vi "CodigoLabView 3.5.vi"() -> (11 "Releb 2":bool)   [LabVIEW 2025]
uses:
  <vilib>/Utility/NIReport.llb/Report Type.ctl
  <vilib>/Instr/_visa.llb/VISA Configure Serial Port (Instr).vi
  <vilib>/addons/_office/excel.llb/Excel Easy Table (str).vi
  <vilib>/Utility/NIReport.llb/NI_report.lvclass
  <vilib>/addons/_office/NI_ReportGenerationToolkit.lvlib
  <vilib>/Utility/NIReport.llb/NI_ReportGenerationCore.lvlib
  <vilib>/Utility/NIReport.llb/Excel/NI_Excel.lvclass
panel:
  out "errorout":errorcluster
  out "Vrno":refnum<visa-resource-name>
  out "Texto":path=path "C:/Users/Lucas Navarro/Desktop/Ruka/ME2/pf/Jamon.txt"
  out "Historial Tensión de Línea":dbl[](graph)
  out "Historial Tomacorriente 4":dbl[](graph)
  out "Historial Tomacorriente 3":dbl[](graph)
  out "Historial Tomacorriente 2":dbl[](graph)
  out "Historial Tomacorriente 1":dbl[](graph)
  in  "?":bool
  in  "RUTA DE REGISTRO":path
  out "NP4":dbl(knob) scale=0.0..100.0
  out "NP3":dbl(knob) scale=0.0..100.0
  out "NP2":dbl(knob) scale=0.0..100.0
  out "R ON 4":bool
  out "R ON 3":bool
  out "R ON 2":bool
  out "ST":string
  out "R ON 1":bool
  out "NT":dbl(knob) scale=100.0..300.0
  out "NP1":dbl(knob) scale=0.0..100.0
  out "Releb 4":bool
  out "Relea 4":bool
  out "Rele 4":bool
  out "T4":bool
  out "Estado 4":string
  in  "Relé N°4":bool
  out "SP4":string
  out "Releb 3":bool
  out "Relea 3":bool
  out "Rele 3":bool
  out "T3":bool
  out "Estado 3":string
  out "SP3":string
  in  "Relé N°3":bool
  out "Relea 2":bool
  out "Rele 2":bool
  out "T2":bool
  out "Estado 2":string
  out "SP2":string
  in  "Relé N°2":bool
  out "Releb 1":bool
  out "Relea 1":bool
  out "Rele 1":bool
  out "T1":bool
  out "Estado 1":string
  out "SP1":string
  in  "Relé N°1":bool
  in  "PUERTO DE COMUNICACIÓN":refnum<visa-resource-name>
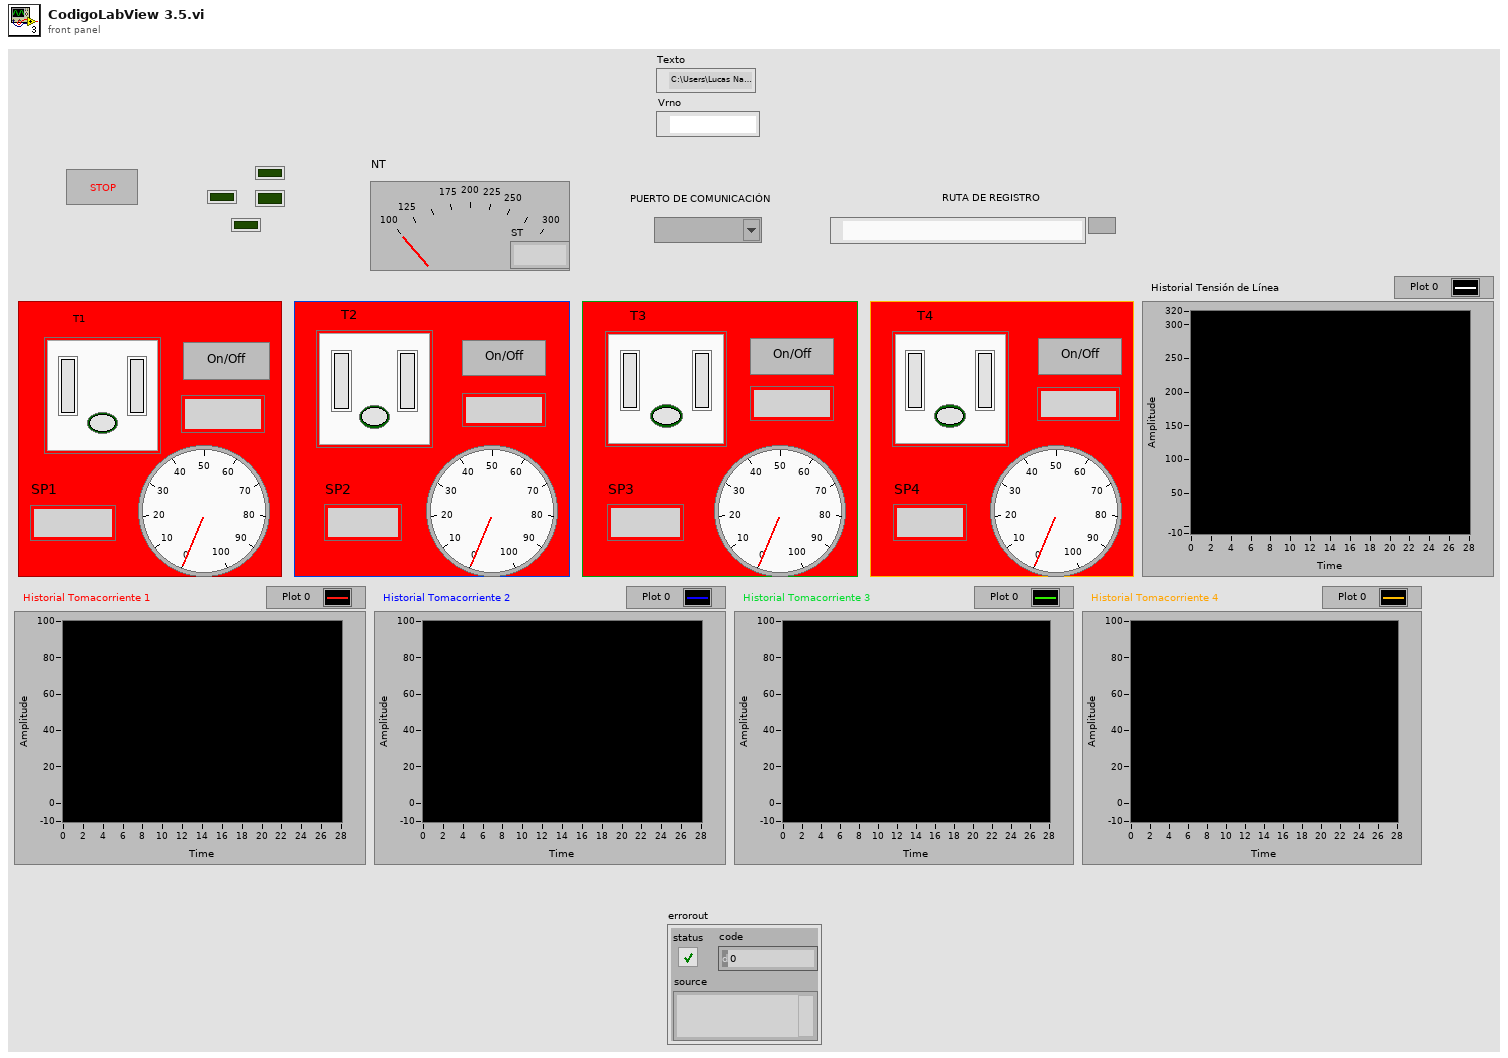
[diagram p1: front panel]
types:
  T1 = typedef "NI_ReportGenerationCore.lvlib/Report Type.ctl" = enum16{"HTML", "Word", "Excel"}
  T2 = cluster{"W1":string, "W2":string, "W3":string, "W4":string, "V":string}
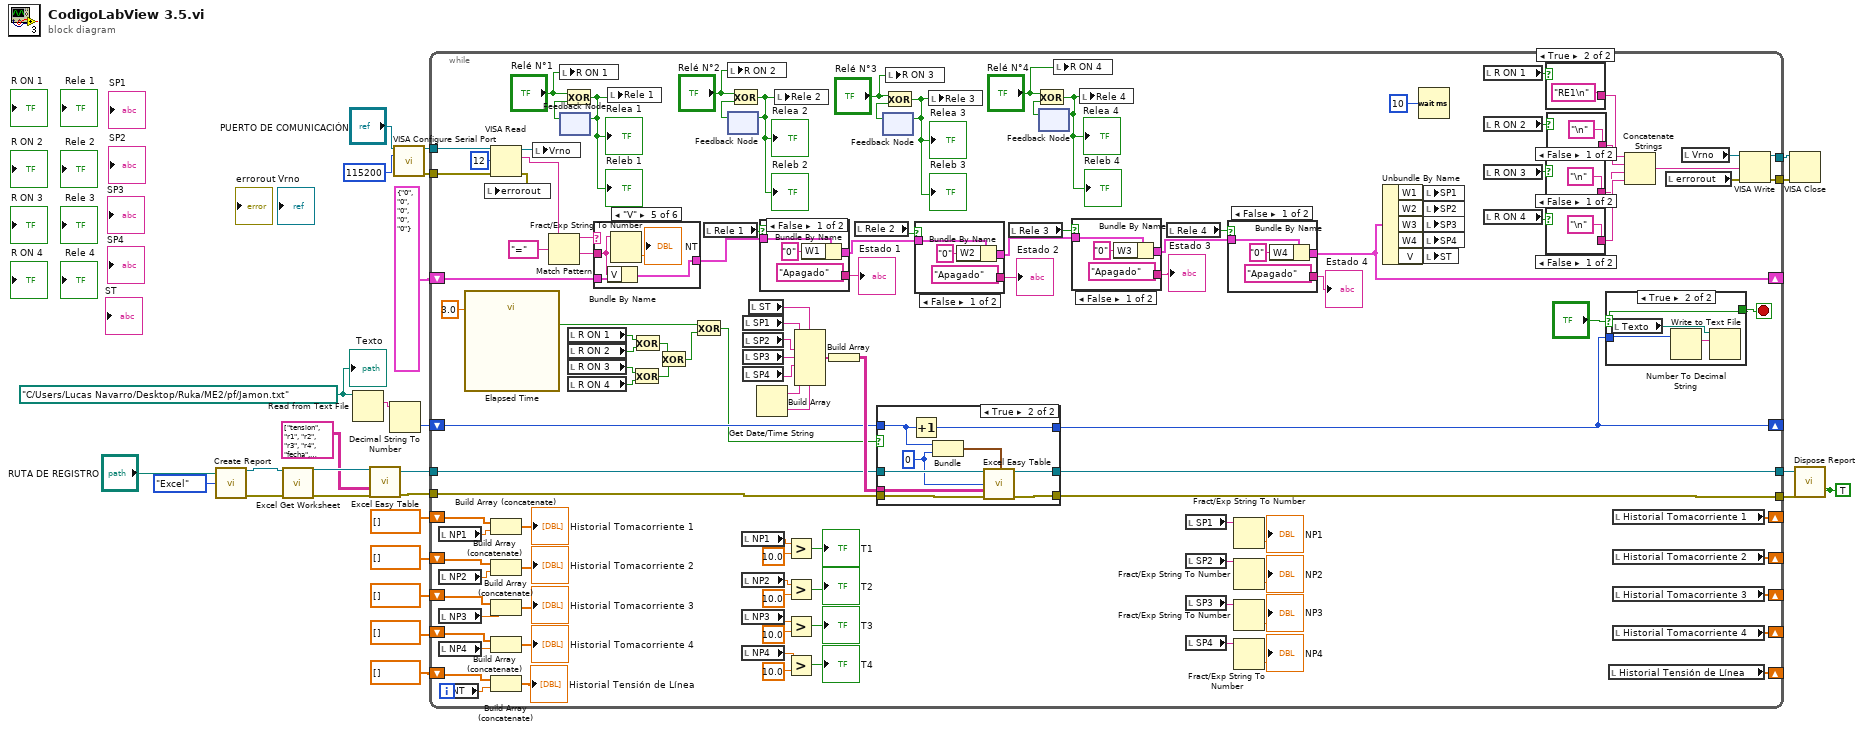
[diagram p0: block diagram]
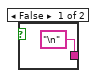
[diagram p2: hidden frame]
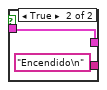
[diagram p3: hidden frame]
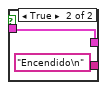
[diagram p4: hidden frame]
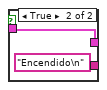
[diagram p5: hidden frame]
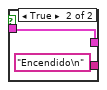
[diagram p8: hidden frame]
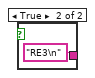
[diagram p9: hidden frame]
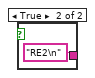
[diagram p10: hidden frame]
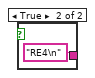
[diagram p11: hidden frame]
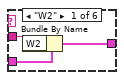
[diagram p12: hidden frame]
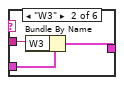
[diagram p13: hidden frame]
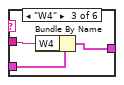
[diagram p14: hidden frame]
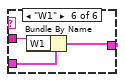
[diagram p16: hidden frame]
diagram:
  w2 = path "C:/Users/Lucas Navarro/Desktop/Ruka/ME2/pf/Jamon.txt" ("file (use dialog)")
  w1 = TRUE ("close report? (T)")
  n1 = call <vilib>:"Create Report.vi"("report type"=Report_Type."Excel", "template (empty)"="RUTA DE REGISTRO") -> ("report out"=w18:refnum<class "NI_report.lvclass">, "error out"=w17:errorcluster)  [unwired: 12 in]
  n2 = call <vilib>:"Excel Get Worksheet.vi"("report in"=w18, "error in (no error)"=w17) -> ("report out"=w16:refnum<class "NI_report.lvclass">, "error out"=w15:errorcluster)  [unwired: 12 in]
  n3 = Read from Text File(file (use dialog)=w2) -> (text=w9:string)  [unwired: 3 in, 3 out]
  n4 = call-poly <vilib>:"Excel Easy Table.vi"("report in"=w16, "text data"=string[][] [["tension", "r1", "r2", "r3", "r4", "fecha", "hora"]], "error in (no error)"=w15) -> ("report out"=w13:refnum<class "NI_report.lvclass">, "error out"=w12:errorcluster)  [unwired: 8 in, 3 out]
  n5 = Decimal String To Number(string=w9) -> (number=w8:i32)  [unwired: 2 in, 1 out]
  n6 = call-poly "VISA Configure Serial Port"("VISA resource name"="PUERTO DE COMUNICACIÓN", "baud rate (9600)"=u32 115200) -> ("VISA resource name out"=w27:refnum<visa-resource-name>, "error out"=w24:errorcluster)  [unwired: 12 in]
  n7 = while {
    tunnel: w27 -> [w127]
    tunnel: w24 -> [w126]
    shift-right: [w75] -> _
    shift-left: T2 {"W1"="0", "W2"="0", "W3"="0", "W4"="0", "V"="0"} -> [w74]
    tunnel: [w129] -> w22
    tunnel: [w128] -> w21
    shift-right: [w84] -> _
    shift-left: w8 -> [w97]
    tunnel: w13 -> [w118]
    tunnel: w12 -> [w117]
    tunnel: [w110] -> w11
    tunnel: [w109] -> w10
    shift-right: [w31] -> _
    shift-left: dbl[] [] ("array") -> [w106]
    shift-right: [w32] -> _
    shift-left: dbl[] [] ("array") -> [w105]
    shift-right: [w33] -> _
    shift-left: dbl[] [] ("array") -> [w104]
    shift-right: [w35] -> _
    shift-left: dbl[] [] ("array") -> [w103]
    shift-right: [w34] -> _
    shift-left: dbl[] [] ("array") -> [w102]
    stop <- w107 stop-if-true
    n8 = local read "NP1"() -> (w57:dbl)
    n9 = local read "NP2"() -> (w56:dbl)
    n10 = local read "NP3"() -> (w55:dbl)
    n11 = local read "NP4"() -> (w54:dbl)
    n12 = local read "NT"() -> (w53:dbl)
    n13 = call "Elapsed Time"("Time Target (s)"=3.0) -> ("Time has Elapsed"=w29:bool)  [unwired: 11 in, 7 out]
    n14 = VISA Read(VISA resource name=w127, byte count=u32 12 ("Bytes at Port"), error in (no error)=w126) -> (VISA resource name out=w79:refnum<visa-resource-name>, read buffer=w73:string, error out=w78:errorcluster)  [unwired: 1 out]
    n15 = local write "errorout"(w78) -> ()
    n16 = Build Array (concatenate)(w106, w57) -> (→"Historial Tomacorriente 1":dbl[])
    n17 = Build Array (concatenate)(w105, w56) -> (→"Historial Tomacorriente 2":dbl[])
    n18 = Build Array (concatenate)(w104, w55) -> (→"Historial Tomacorriente 3":dbl[])
    n19 = Build Array (concatenate)(w103, w54) -> (→"Historial Tomacorriente 4":dbl[])
    n20 = Build Array (concatenate)(w102, w53) -> (→"Historial Tensión de Línea":dbl[])
    n21 = local write "Vrno"(w79) -> ()
    n22 = Match Pattern(string=w73, regular expression="=") -> (before substring=w146:string, after substring=w131:string)  [unwired: 1 in, 2 out]
    n23 = local write "R ON 1"("Relé N°1") -> ()
    n24 = feedback #1() -> (w145:bool)  [unwired: 1 in]
    n25 = Exclusive Or(1:w145, 2:"Relé N°1") -> (0:w83:bool)
    "Releb 1" <- w83
    "Relea 1" <- w83
    n26 = feedback-in #1(w83) -> ()
    n27 = local read "R ON 1"() -> (w116:bool)
    n28 = local read "R ON 2"() -> (w115:bool)
    n29 = local read "R ON 3"() -> (w113:bool)
    n30 = local read "R ON 4"() -> (w114:bool)
    n31 = case shown="\"V\"" w146 {
      tunnel: w131 -> [w197 w200 w203 _ w208 w211]
      tunnel: w74 -> [w199 w202 w205 w206 w210 w213]
      tunnel: [w198 w201 w204 w206 w209 w212] -> w125
      frame "W2" {
        n32 = Bundle By Name(cluster=w199, "W2"=w197) -> (w198:T2)
      }
      frame "W3" {
        n33 = Bundle By Name(cluster=w202, "W3"=w200) -> (w201:T2)
      }
      frame "W4" {
        n34 = Bundle By Name(cluster=w205, "W4"=w203) -> (w204:T2)
      }
      frame "False", Default {
      }
      frame "V" {
        n35 = Bundle By Name(cluster=w210, "V"=w208) -> (w209:T2)
        n36 = Fract/Exp String To Number(string=w208) -> (number=→"NT":dbl)  [unwired: 3 in, 1 out]
      }
      frame "W1" {
        n37 = Bundle By Name(cluster=w213, "W1"=w211) -> (w212:T2)
      }
    }
    n38 = local write "Rele 1"(w83) -> ()
    n39 = Exclusive Or(1:w114, 2:w113) -> (0:w112:bool)
    n40 = Exclusive Or(1:w115, 2:w116) -> (0:w111:bool)
    n41 = Exclusive Or(1:w112, 2:w111) -> (0:w28:bool)
    n42 = Exclusive Or(1:w28, 2:w29) -> (0:w30:bool)
    n43 = local read "Rele 1"() -> (w124:bool)
    n44 = local write "R ON 2"("Relé N°2") -> ()
    n45 = feedback #2() -> (w139:bool)  [unwired: 1 in]
    n46 = Exclusive Or(1:w139, 2:"Relé N°2") -> (0:w82:bool)
    "Releb 2" <- w82
    "Relea 2" <- w82
    n47 = feedback-in #2(w82) -> ()
    n48 = local read "NP1"() -> (w52:dbl)
    n49 = local read "NP2"() -> (w51:dbl)
    n50 = local read "NP3"() -> (w50:dbl)
    n51 = local read "NP4"() -> (w49:dbl)
    n52 = local read "SP1"() -> (w61:string)
    n53 = local read "SP2"() -> (w60:string)
    n54 = local read "SP3"() -> (w59:string)
    n55 = local read "SP4"() -> (w58:string)
    n56 = local read "ST"() -> (w62:string)
    n57 = Get Date/Time String() -> (date string=w122:string, time string=w123:string)  [unwired: 3 in]
    n58 = case shown="False" w124 {
      tunnel: w125 -> [w187 w190]
      tunnel: [w186 w190] -> w95
      tunnel: ["Apagado" "Encendido\n"] -> w88
      frame False {
        n59 = Bundle By Name(cluster=w187, "W1"="0") -> (w186:T2)
      }
      frame True {
      }
    }
    "Estado 1" <- w88
    n60 = local write "Rele 2"(w82) -> ()
    n61 = Greater?(x=w52, y=10.0) -> (0:→"T1":bool)
    n62 = Greater?(x=w51, y=10.0) -> (0:→"T2":bool)
    n63 = Greater?(x=w50, y=10.0) -> (0:→"T3":bool)
    n64 = Greater?(x=w49, y=10.0) -> (0:→"T4":bool)
    n65 = Build Array(w62, w61, w60, w59, w58, w122, w123) -> (w120:string[])
    n66 = Build Array(w120) -> (w121:string[][])
    n67 = local read "Rele 2"() -> (w92:bool)
    n68 = case shown="True" w30 {
      tunnel: w121 -> [_ w184]
      tunnel: w117 -> [w175 w183]
      tunnel: [w174 w182] -> w110
      tunnel: [w175 w181] -> w109
      tunnel: w118 -> [w174 w180]
      tunnel: w97 -> [w173 w179]
      tunnel: [w173 w178] -> w84
      frame False {
      }
      frame True {
        w176 = 0 ("iteration")
        n69 = Increment(x=w179) -> (x+1=w178:i32)
        n70 = Bundle(w179, "iteration"=w176) -> (w177:cluster{i32, "iteration":i32})  [unwired: 1 in]
        n71 = call-poly <vilib>:"Excel Easy Table.vi"("report in"=w180, "iteration"=w176, "start (0, 0)"=w177, "text data"=w184, "error in (no error)"=w183) -> ("report out"=w182:refnum<class "NI_report.lvclass">, "error out"=w181:errorcluster)  [unwired: 6 in, 3 out]
      }
    }
    n72 = feedback #3() -> (w137:bool)  [unwired: 1 in]
    n73 = Exclusive Or(1:w137, 2:"Relé N°3") -> (0:w81:bool)
    "Relea 3" <- w81
    "Releb 3" <- w81
    n74 = feedback-in #3(w81) -> ()
    n75 = local write "R ON 3"("Relé N°3") -> ()
    n76 = case shown="False" w92 {
      tunnel: w95 -> [w165 w168]
      tunnel: [w164 w168] -> w94
      tunnel: ["Apagado" "Encendido\n"] -> w86
      frame False {
        n77 = Bundle By Name(cluster=w165, "W2"="0") -> (w164:T2)
      }
      frame True {
      }
    }
    "Estado 2" <- w86
    n78 = local write "Rele 3"(w81) -> ()
    n79 = local read "Rele 3"() -> (w91:bool)
    n80 = feedback #4() -> (w135:bool)  [unwired: 1 in]
    n81 = Exclusive Or(1:w135, 2:"Relé N°4") -> (0:w80:bool)
    "Relea 4" <- w80
    "Releb 4" <- w80
    n82 = feedback-in #4(w80) -> ()
    n83 = local write "R ON 4"("Relé N°4") -> ()
    n84 = case shown="False" w91 {
      tunnel: w94 -> [w159 w162]
      tunnel: [w158 w162] -> w93
      tunnel: ["Apagado" "Encendido\n"] -> w87
      frame False {
        n85 = Bundle By Name(cluster=w159, "W3"="0") -> (w158:T2)
      }
      frame True {
      }
    }
    "Estado 3" <- w87
    n86 = local write "Rele 4"(w80) -> ()
    n87 = local read "Rele 4"() -> (w90:bool)
    n88 = local read "SP1"() -> (w66:string)
    n89 = local read "SP2"() -> (w64:string)
    n90 = local read "SP3"() -> (w63:string)
    n91 = local read "SP4"() -> (w65:string)
    n92 = case shown="False" w90 {
      tunnel: w93 -> [w153 w156]
      tunnel: [w152 w156] -> w75
      tunnel: ["Apagado" "Encendido\n"] -> w89
      frame False {
        n93 = Bundle By Name(cluster=w153, "W4"="0") -> (w152:T2)
      }
      frame True {
      }
    }
    "Estado 4" <- w89
    n94 = Fract/Exp String To Number(string=w66) -> (number=→"NP1":dbl)  [unwired: 3 in, 1 out]
    n95 = Fract/Exp String To Number(string=w64) -> (number=→"NP2":dbl)  [unwired: 3 in, 1 out]
    n96 = Fract/Exp String To Number(string=w63) -> (number=→"NP3":dbl)  [unwired: 3 in, 1 out]
    n97 = Fract/Exp String To Number(string=w65) -> (number=→"NP4":dbl)  [unwired: 3 in, 1 out]
    n98 = Unbundle By Name(w75) -> ("W1"=w101:string, "W2"=w98:string, "W3"=w99:string, "W4"=w100:string, "V"=w96:string)
    n99 = Wait (ms)(milliseconds to wait=u32 10) -> ()  [unwired: 1 out]
    n100 = local write "SP1"(w101) -> ()
    n101 = local write "SP2"(w98) -> ()
    n102 = local write "SP3"(w99) -> ()
    n103 = local write "SP4"(w100) -> ()
    n104 = local write "ST"(w96) -> ()
    n105 = local read "R ON 1"() -> (w68:bool)
    n106 = local read "R ON 2"() -> (w142:bool)
    n107 = local read "R ON 3"() -> (w141:bool)
    n108 = local read "R ON 4"() -> (w143:bool)
    n109 = case shown="True" w68 {
      tunnel: ["\n" "RE1\n"] -> w67
      frame False {
      }
      frame True {
      }
    }
    n110 = case shown="False" w141 {
      tunnel: ["\n" "RE3\n"] -> w132
      frame False {
      }
      frame True {
      }
    }
    n111 = case shown="False" w143 {
      tunnel: ["\n" "RE4\n"] -> w133
      frame False {
      }
      frame True {
      }
    }
    n112 = case shown="False" w142 {
      tunnel: ["\n" "RE2\n"] -> w134
      frame False {
      }
      frame True {
      }
    }
    n113 = case shown="True" "?" {
      selector: "?" -> [_ w171]
      tunnel: w84 -> [_ w172]
      tunnel: [_ w171] -> w107
      frame False {
      }
      frame True {
        n114 = local read "Texto"() -> (w169:path)
        n115 = Number To Decimal String(number=w172) -> (decimal integer string=w170:string)  [unwired: 1 in]
        n116 = Write to Text File(file (use dialog)=w169, text=w170) -> ()  [unwired: 2 in, 3 out]
      }
    }
    n117 = local read "Historial Tensión de Línea"() -> (w34:dbl[])
    n118 = local read "Historial Tomacorriente 1"() -> (w31:dbl[])
    n119 = local read "Historial Tomacorriente 2"() -> (w32:dbl[])
    n120 = local read "Historial Tomacorriente 3"() -> (w33:dbl[])
    n121 = local read "Historial Tomacorriente 4"() -> (w35:dbl[])
    n122 = Concatenate Strings(w67, w134, w132, w133) -> (w130:string)
    n123 = local read "errorout"() -> (w77:errorcluster)
    n124 = local read "Vrno"() -> (w76:refnum<visa-resource-name>)
    n125 = VISA Write(VISA resource name=w76, write buffer=w130, error in (no error)=w77) -> (VISA resource name out=w129:refnum<visa-resource-name>, error out=w128:errorcluster)  [unwired: 1 out]
  }
  n126 = VISA Close(VISA resource name=w22, error in (no error)=w21) -> ()  [unwired: 1 out]
  n127 = call-dynamic "Dispose Report.vi"("report in"=w11, "save changes? (F)"=w1, "error in (no error)"=w10, "close report? (T)"=w1) -> ()  [unwired: 11 in, 1 out]
  "Texto" <- w2
